vi "Abrir-Camera.vi"(0 "Interface Name":string="cam1", 7 "error in":errorcluster) -> (20 "Image Out":T1(plugin-control), 27 "error out":errorcluster)   [LabVIEW 2020]
doc: "Creates, and edits acquisitions using the NI Vision Acquisition Express VI.\n\nThe NI Vision Acquisition Wizard is launched by placing the Express VI on the block diagram. Select an acquisition source and configure an acquisition using NI-IMAQ, NI-IMAQdx, or simulate an acquisition by reading an AVI or image files from a folder. After an acquisition is configured, select controls and indicators to be able to programmatically set in LabVIEW. Double-click the Vision Acquisition Express VI to edit the acquisition.\n\nNote: Any images created by the Express VI need to be disposed after use. Use the IMAQ Dispose.vi to cleanup the images output by the Express VI when they are no longer needed."
uses:
  <vilib>/vision/driver/NI_Vision_Acquisition_Software.lvlib
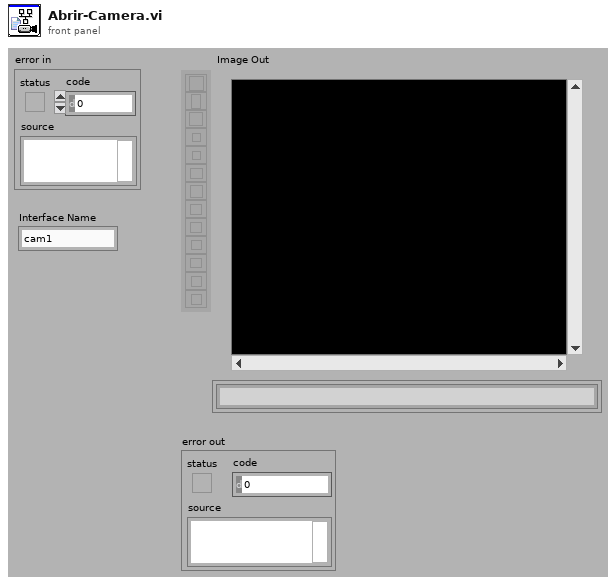
[diagram p1: front panel]
types:
  T1 = typedef "IMAQ Image.ctl" = refnum<image>
  T2 = typedef "IMAQdx.ctl" = refnum<k21>
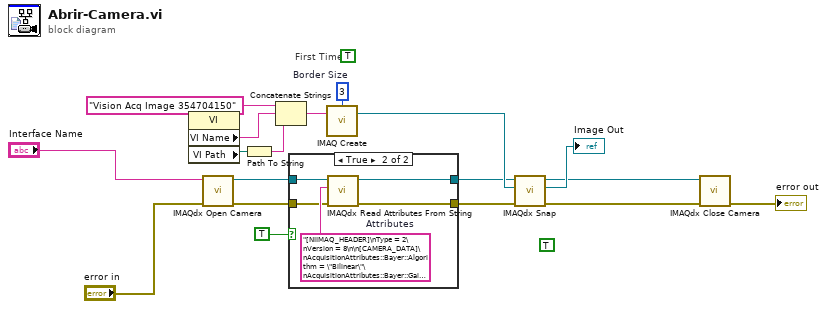
[diagram p0: block diagram]
diagram:
  (unwired) TRUE
  w7 = 3  # Border Size
  (unwired) TRUE
  # "First Time"
  n1 = property class="VI"() -> ("VI Name"=w15:string, "VI Path"=w16:path)  [unwired: 2 in, 2 out]
  n2 = call <vilib>:"IMAQdx Open Camera.vi"("error in"="error in", "Session In"="Interface Name") -> ("error out"=w10:errorcluster, "Session Out"=w11:T2)  [unwired: 1 in, 7 out]
  n3 = Path To String(path=w16) -> (string=w14:string)
  n4 = Concatenate Strings("Vision Acq Image 354704150" ("Image Name"), w15, w14) -> (w12:string)
  n5 = case shown="True" TRUE ("Init Attributes") {
    tunnel: w11 -> [w20 w25]
    tunnel: w10 -> [w19 w23]
    tunnel: [w20 w22] -> w3
    tunnel: [w19 w21] -> w9
    frame False {
    }
    frame True {
      w24 = "[NIIMAQ_HEADER]\nType = 2\nVersion = 8\n\n[CAMERA_DATA]\nAcquisitionAttributes::Bayer::Algorithm = \"Bilinear\"\nAcquisitionAttributes::Bayer::GainB = \"1\"\nAcquisitionAttributes::Bayer::GainG = \"1\"\nAcquisitionAttributes::Bayer::GainR = \"1\"\nAcquisitionAttributes::Bayer::Pattern = \"Use hardware value\"\nAcquisitionAttributes::BitsPerPixel = \"Use hardware value\"\nAcquisitionAttributes::HardwareMaximumQueuedBufferCount = \"1000\"\nAcquisitionAttributes::HardwareRequeueBufferListThreshold = \"50\"\nAcquisitionAttributes::IgnoreFirstFrame = \"false\"\nAcquisitionAttributes::ImageDecoderCopyMode = \"Auto\"\nAcquisitionAttributes::OutputImageType = \"Auto\"\nAcquisitionAttributes::OverwriteMode = \"Get Newest\"\nAcquisitionAttributes::PixelSignedness = \"Use hardware value\"\nAcquisitionAttributes::ReceiveTimestampMode = \"None\"\nAcquisitionAttributes::ShiftPixelBits = \"false\"\nAcquisitionAttributes::SwapPixelBytes = \"false\"\nAcquisitionAttributes::Timeout = \"5000\"\nAcquisitionAttributes::VerticalMirror = \"false\"\nAcquisitionAttributes::VideoMode = \"2304x1536 YUY2 2.00fps\"\nCameraAttributes::BacklightCompensation::Mode = \"Manual\"\nCameraAttributes::BacklightCompensation::Value = \"false\"\nCameraAttributes::Brightness::Mode = \"Manual\"\nCameraAttributes::Brightness::Value = \"128\"\nCameraAttributes::Contrast::Mode = \"Manual\"\nCameraAttributes::Contrast::Value = \"1.28000000000000003\"\nCameraAttributes::Exposure::Mode = \"Manual\"\nCameraAttributes::Exposure::Value = \"0.015625\"\nCameraAttributes::Focus::Mode = \"Manual\"\nCameraAttributes::Focus::Value = \"30\"\nCameraAttributes::Gain::Mode = \"Manual\"\nCameraAttributes::Gain::Value = \"0\"\nCameraAttributes::Pan::Mode = \"Manual\"\nCameraAttributes::Pan::Value = \"0\"\nCameraAttributes::Saturation::Mode = \"Manual\"\nCameraAttributes::Saturation::Value = \"128\"\nCameraAttributes::Sharpness::Mode = \"Manual\"\nCameraAttributes::Sharpness::Value = \"128\"\nCameraAttributes::Tilt::Mode = \"Manual\"\nCameraAttributes::Tilt::Value = \"0\"\nCameraAttributes::WhiteBalance::Mode = \"Auto\"\nCameraAttributes::Zoom::Mode = \"Manual\"\nCameraAttributes::Zoom::Value = \"100\"\n"  # Attributes
      n6 = call <vilib>:"IMAQdx Read Attributes From String.vi"("error in"=w23, "Attributes String In"=w24, "Session In"=w25) -> ("error out"=w21:errorcluster, "Session Out"=w22:T2)  [unwired: 7 out]
    }
  }
  n7 = call "IMAQ Create"("Border Size"=w7, "Image Name"=w12) -> ("New Image"=w4:T1)  [unwired: 2 in, 2 out]
  n8 = call <vilib>:"IMAQdx Snap.vi"("error in"=w9, "Image In"=w4, "Session In"=w3) -> ("error out"=w6:errorcluster, "Image Out"=→"Image Out":T1, "Session Out"=w1:T2)  [unwired: 6 out]
  n9 = call <vilib>:"IMAQdx Close Camera.vi"("error in"=w6, "Session In"=w1) -> ("error out"=→"error out":errorcluster)  [unwired: 9 out]
